vi "VI-Find Project Item (lib).vi"(0 "Library Refnum":refnum<vi>, 5 "Type":string, 7 "Name":string, 11 "error in (no error)":errorcluster) -> (4 "reference out":refnum<vi>, 6 "ProjectItem":refnum<vi>, 8 "Found":bool, 15 "error out":errorcluster)   [LabVIEW 2020]
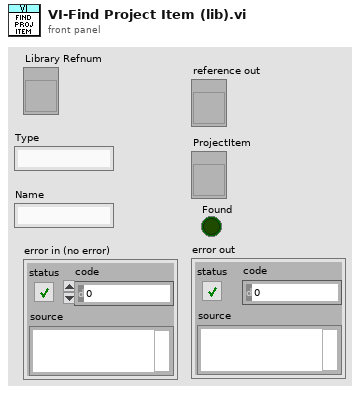
[diagram p1: front panel]
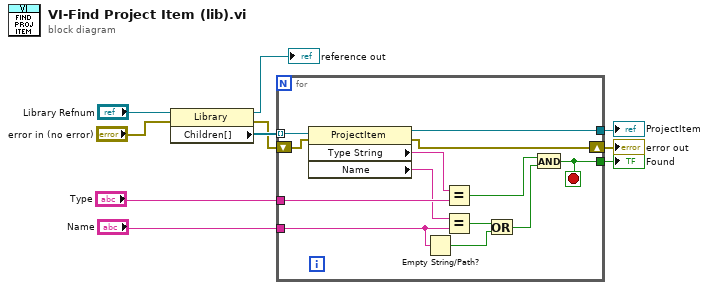
[diagram p0: block diagram]
diagram:
  n1 = property class="Library"(reference="Library Refnum", error in="error in (no error)") -> (reference out=→"reference out":refnum<vi>, error out=w5:errorcluster, "Children[]"=w7:refnum<vi>[])
  n2 = for {
    tunnel: w7 -> [w23] mode=indexing
    tunnel: [w20] -> w8
    tunnel: "Type" -> [w19]
    tunnel: "Name" -> [w12]
    tunnel: [w18] -> w1
    shift-right: [w16] -> w4
    shift-left: w5 -> [w17]
    stop <- w18 stop-if-true
    n3 = property class="ProjectItem"(reference=w23, error in=w17) -> (reference out=w20:refnum<vi>, error out=w16:errorcluster, "Type String"=w13:string, "Name"=w11:string)
    n4 = Empty String/Path?(string/path=w12) -> (empty?=w14:bool)
    n5 = Equal?(x=w13, y=w19) -> (x = y?=w22:bool)
    n6 = Equal?(x=w11, y=w12) -> (x = y?=w21:bool)
    n7 = Or(x=w21, y=w14) -> (x .or. y?=w15:bool)
    n8 = And(x=w22, y=w15) -> (x .and. y?=w18:bool)
  }
  "ProjectItem" <- w8
  "error out" <- w4
  "Found" <- w1
